vi "simFPGA.vi"() -> ()   [LabVIEW 2014]
panel:
  in  "milliseconds to wait":u32
  out "Waveform Chart":dbl(graph)
  out "k3":dbl
  out "k2":u32
  in  "stop":bool
  in  "k1 [count/ms]":u16
  in  "freq":u8
  out "Waveform Graph":dbl[](graph)
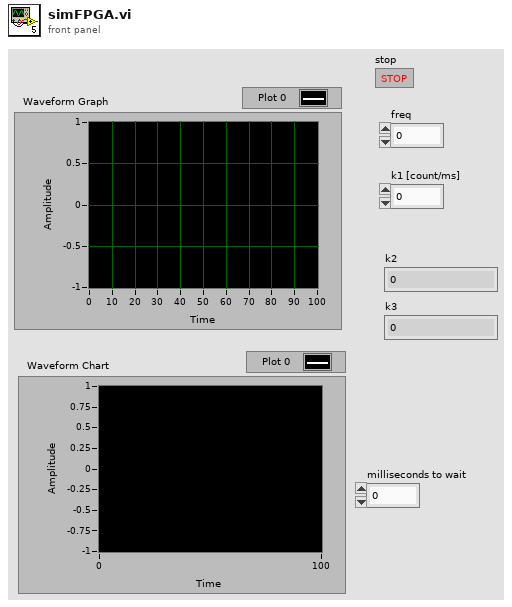
[diagram p1: front panel]
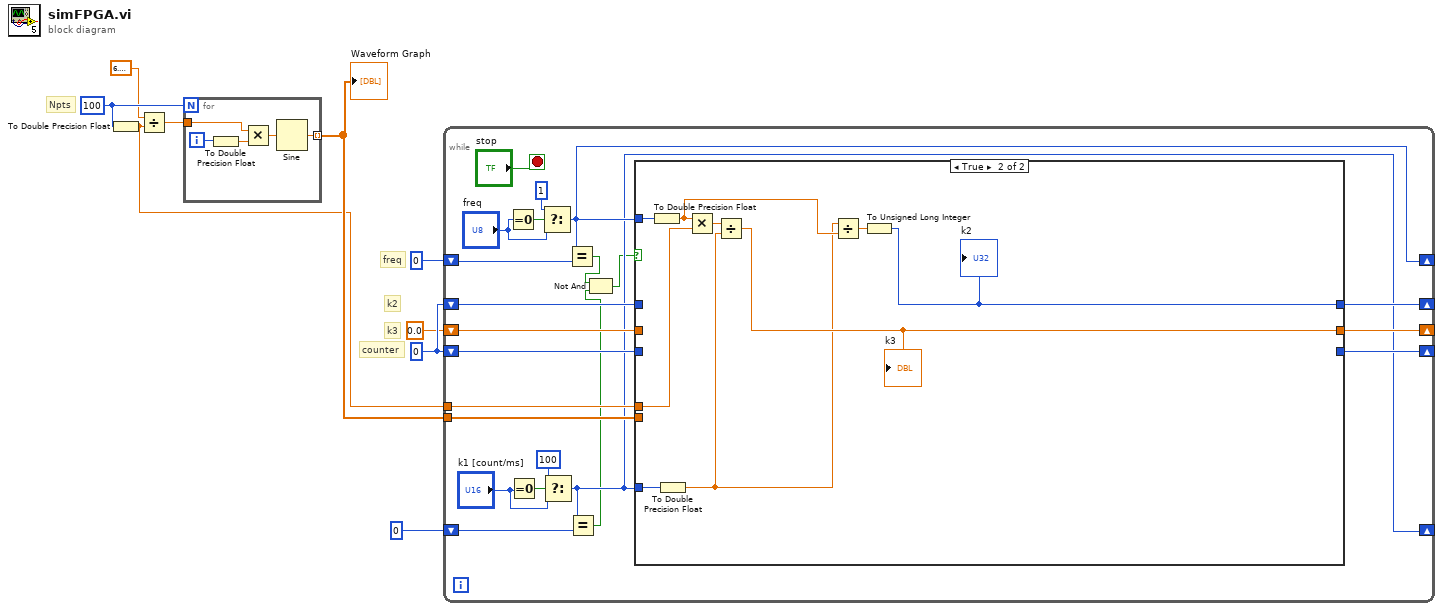
[diagram p0: block diagram]
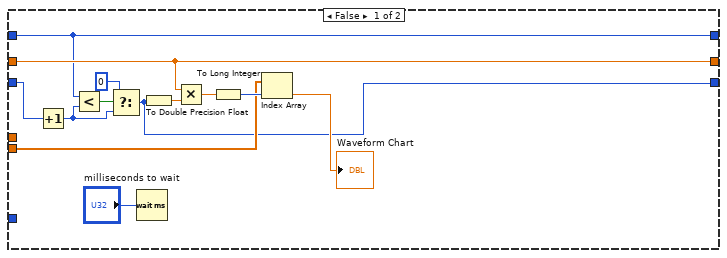
[diagram p2: hidden frame]
diagram:
  w3 = u32 0
  w9 = 100
  # "k2"
  # "k3"
  # "counter"
  # "freq"
  # "Npts"
  n1 = To Double Precision Float(number=w9) -> (double precision float=w5:dbl)
  n2 = Divide(x=6.283185307179586, y=w5) -> (x/y=w8:dbl)
  n3 = for {
    N: w9 -> [_]
    tunnel: w8 -> [w11]
    tunnel: [w12] -> w6 mode=indexing
    i -> [w14]
    n4 = To Double Precision Float(number=w14) -> (double precision float=w13:dbl)
    n5 = Multiply(x=w11, y=w13) -> (x*y=w10:dbl)
    n6 = Sine(x=w10) -> (sin(x)=w12:dbl)
  }
  "Waveform Graph" <- w6
  n7 = while {
    tunnel: w6 -> [w30]
    tunnel: w5 -> [w29]
    shift-right: [w31] -> _
    shift-left: u8 0 -> [w34]
    shift-right: [w23] -> _
    shift-left: w3 -> [w28]
    shift-right: [w24] -> _
    shift-left: 0.0 -> [w27]
    shift-right: [w25] -> _
    shift-left: w3 -> [w26]
    shift-right: [w18] -> _
    shift-left: u16 0 -> [w20]
    stop <- "stop" stop-if-true
    n8 = Equal To 0?(x="freq") -> (x = 0?=w35:bool)
    n9 = Equal To 0?(x="k1 [count/ms]") -> (x = 0?=w22:bool)
    n10 = Select(t=u8 1, s=w35, f="freq") -> (s? t:f=w31:u8)
    n11 = Select(t=u16 100, s=w22, f="k1 [count/ms]") -> (s? t:f=w18:u16)
    n12 = Equal?(x=w31, y=w34) -> (x = y?=w17:bool)
    n13 = Equal?(x=w18, y=w20) -> (x = y?=w16:bool)
    n14 = Not And(1:w16, 2:w17) -> (0:w15:bool)
    n15 = case shown="True" w15 {
      tunnel: w31 -> [_ w58]
      tunnel: w30 -> [w41 _]
      tunnel: w29 -> [_ w57]
      tunnel: w28 -> [w46 _]
      tunnel: w27 -> [w44 _]
      tunnel: w26 -> [w37 _]
      tunnel: [w37 w52] -> w25
      tunnel: [w44 w55] -> w24
      tunnel: [w38 _] -> w23
      tunnel: w18 -> [_ w51]
      frame False {
        n16 = Increment(x=w46) -> (x+1=w48:u32)
        n17 = Less?(x=w37, y=w48) -> (x < y?=w49:bool)
        n18 = Select(t=u32 0, s=w49, f=w48) -> (s? t:f=w38:u32)
        n19 = Wait (ms)(milliseconds to wait="milliseconds to wait") -> ()  [unwired: 1 out]
        n20 = To Double Precision Float(number=w38) -> (double precision float=w45:dbl)
        n21 = Multiply(x=w44, y=w45) -> (x*y=w42:dbl)
        n22 = To Long Integer(number=w42) -> (32bit integer=w43:i32)
        n23 = Index Array(array=w41, index=w43) -> (element=→"Waveform Chart":dbl)
      }
      frame True {
        n24 = To Double Precision Float(number=w58) -> (double precision float=w54:dbl)
        n25 = To Double Precision Float(number=w51) -> (double precision float=w50:dbl)
        n26 = Multiply(x=w54, y=w57) -> (x*y=w56:dbl)
        n27 = Divide(x=w56, y=w50) -> (x/y=w55:dbl)
        "k3" <- w55
        n28 = Divide(x=w50, y=w54) -> (x/y=w53:dbl)
        n29 = To Unsigned Long Integer(number=w53) -> (unsigned 32bit integer=w52:u32)
        "k2" <- w52
      }
    }
  }
